vi "Main.vi"() -> ()   [LabVIEW 2019]
uses:
  Controls/FGV_State.ctl
panel:
  out "Time has elapsed?":bool
  in  "Start":bool
  out "Elapsed time (s)":dbl=5.0 format="%#_2g"
  in  "Time target (s)":dbl=5.0
  in  "Stop":bool
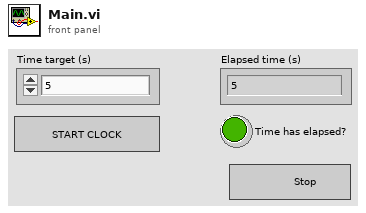
[diagram p1: front panel]
types:
  T1 = typedef "FGV_State.ctl" = enum16{"Read", "Set"}
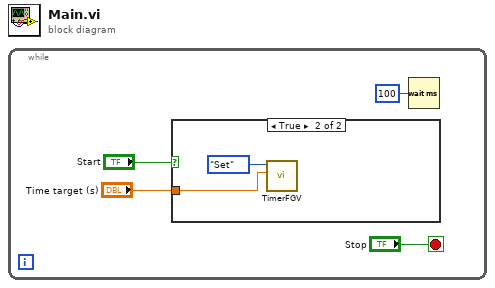
[diagram p0: block diagram]
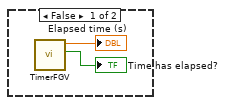
[diagram p2: hidden frame]
diagram:
  n1 = while {
    stop <- "Stop" stop-if-true
    n2 = case shown="True" "Start" {
      tunnel: "Time target (s)" -> [_ w7]
      frame False {
        n3 = call "TimerFGV.vi"() -> ("Time has Elapsed?"=→"Time has elapsed?":bool, "Elapsed Time (s)"=→"Elapsed time (s)":dbl)  [unwired: 10 in]
      }
      frame True {
        n4 = call "TimerFGV.vi"("Time Target (s)"=w7, "FGV State"=FGV_State."Set") -> ()  [unwired: 8 in, 2 out]
      }
    }
    n5 = Wait (ms)(milliseconds to wait=u32 100) -> ()  [unwired: 1 out]
  }
